vi "WriteToGpib.vi"(8 "error in (no error)":errorcluster, 9 "String to Send":string="*idn?", 10 "checksum":bool, 11 "VISA Refnum in":refnum<visa-resource-name>) -> (0 "error out":errorcluster, 3 "VISA Refnum out":refnum<visa-resource-name>)   [LabVIEW 2013]
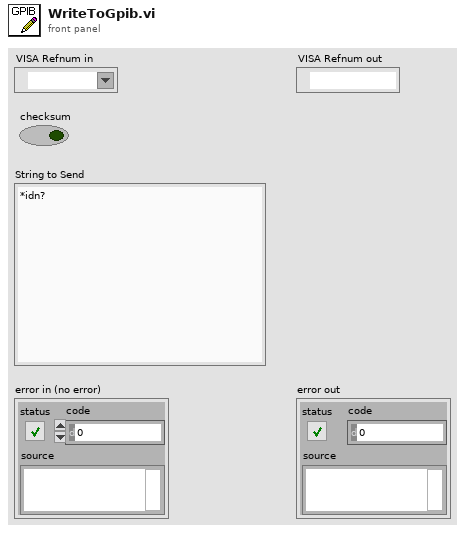
[diagram p1: front panel]
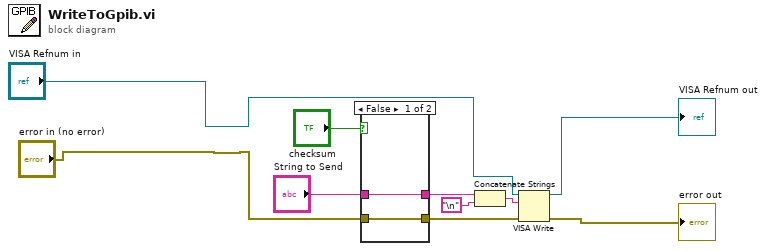
[diagram p0: block diagram]
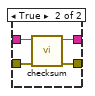
[diagram p2: hidden frame]
diagram:
  n1 = case shown="False" "checksum" {
    tunnel: [w11 w16] -> w4
    tunnel: "error in (no error)" -> [w11 w15]
    tunnel: "String to Send" -> [w12 w14]
    tunnel: [w12 w13] -> w6
    frame False {
    }
    frame True {
      n2 = call "checksum.vi"("error in (no error)"=w15, "Eingabe"=w14) -> ("Error Out"=w16:errorcluster, "Ausgabe"=w13:string)  [unwired: 8 in]
    }
  }
  n3 = Concatenate Strings(w6, "\n") -> (w8:string)
  n4 = VISA Write(VISA resource name="VISA Refnum in", write buffer=w8, error in (no error)=w4) -> (VISA resource name out=→"VISA Refnum out":refnum<visa-resource-name>, error out=→"error out":errorcluster)  [unwired: 1 out]
